vi "AddToLog.vi"(8 "error in (no error)":errorcluster, 11 "Log String":string) -> (0 "error out":errorcluster)   [LabVIEW 2012]
uses:
  Dashboard Global Data.vi
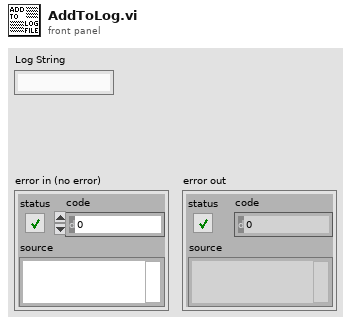
[diagram p1: front panel]
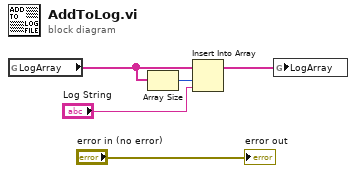
[diagram p0: block diagram]
diagram:
  n1 = global read "Dashboard Global Data.vi" "LogArray"() -> (w1:string[])
  n2 = Array Size(array=w1) -> (size(s)=w5:i32)
  n3 = Insert Into Array(array=w1, index=w5, new element="Log String") -> (w2:string[])
  n4 = global write "Dashboard Global Data.vi" "LogArray"(w2) -> ()
  "error out" <- "error in (no error)"
